vi "macro_AutoHelp_DelayedAction.vi"() -> ()   [LabVIEW 2019, in "Trajectory_Library.lvlib"]
uses:
  Trajectory_Library.lvlib
panel:
  out "Delayed Action Pulse":bool
  out "Delayed Action":bool
  in  "New Step":bool
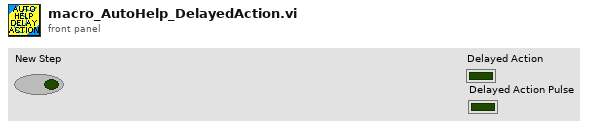
[diagram p1: front panel]
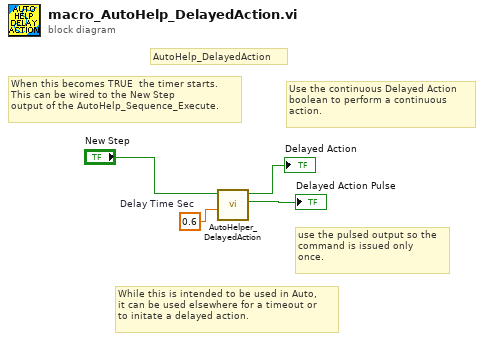
[diagram p0: block diagram]
diagram:
  w4 = 0.6  # Delay Time Sec
  # "AutoHelp_DelayedAction"
  # "While this is intended to be used in Auto, \nit can be used elsewhere for a timeout or\nto initate a delayed action."
  # "Use the continuous Delayed Action\nboolean to perform a continuous \naction."
  # "When this becomes TRUE  the timer starts.  \nThis can be wired to the New Step\noutput of the AutoHelp_Sequence_Execute."
  # "use the pulsed output so the\ncommand is issued only\nonce."
  n1 = call "AutoHelper_DelayedAction.vi"("Delay Time Sec"=w4, "New Step"="New Step") -> ("Delayed Action Pulse"=→"Delayed Action Pulse":bool, "Delayed Action"=→"Delayed Action":bool)  [unwired: 5 in, 3 out]
